vi "SetGearManipulatorOpenClose.vi"(11 "Gear Manipulator Open Close":enum16{"Open", "Close"}(ring)) -> ()   [LabVIEW 2016, in "Gear Manipulator.lvclass"]
uses:
  Gear Manipulator.lvclass
  Gear Manipulator.lvclass/Gear Manipulator.ctl
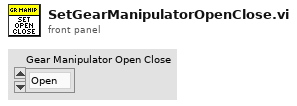
[diagram p1: front panel]
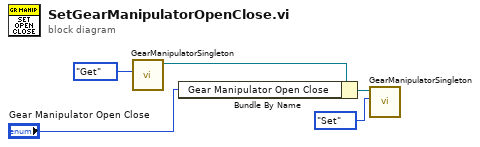
[diagram p0: block diagram]
diagram:
  n1 = call "GearManipulatorSingleton.vi"("Get/Set"=enum16{"Get", "Set"}."Get") -> ("Gear Manipulator.lvclass"=w3:refnum<class "Gear Manipulator.lvclass">)  [unwired: 9 in, 1 out]
  n2 = Bundle By Name(cluster=w3, "Gear Manipulator Open Close"="Gear Manipulator Open Close") -> (w2:refnum<class "Gear Manipulator.lvclass">)
  n3 = call "GearManipulatorSingleton.vi"("Get/Set"=enum16{"Get", "Set"}."Set", "Gear Manipulator.lvclass"=w2) -> ()  [unwired: 8 in, 2 out]
